vi "YaxisSetup.vi"(8 "Mapping":enum8{"Lin", "Log"}(ring), 9 "HeightAxisBounds":T4, 10 "gnuplotIn":string) -> (2 "gnuplotOut":string)   [LabVIEW 2013]
uses:
  minAndMax.ctl
  AutoManualNumber.ctl
  ticsAndGrids.ctl
  tics.ctl
  grids.ctl
  axisName.ctl
panel:
  in  "Post-setup overrides":string="set ytics format '\\color{g}$%g$' offset 0.8,0\nset ylabel '\\color{g}{$h$ (mm)}' offset 12.8\t# Big offset required as format string makes Ytics look longer than they are"
  in  "HeightTicsAndGrids":T1={"tics"={"ticMin"=10.0, "ticStep"=0.0, "ticMax"=1000.0, "minorDivsPerMajor"=10, "ticSpacing"=enum."Auto Tics", "ticPosition"=enum."Outside, no mirror"}, "Grids"={"Gridlines"=enum."Major and Minor", "Zeroaxis"=enum."No zero axis"}, "Mapping"=enum."Lin"}
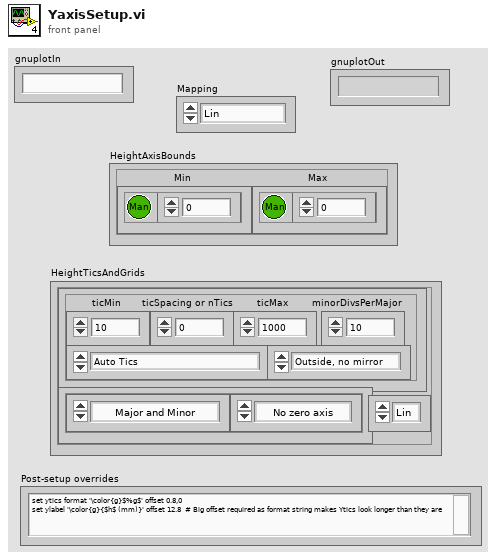
[diagram p1: front panel]
types:
  T1 = typedef "ticsAndGrids.ctl" = cluster{"tics":T2, "Grids":T3, "Mapping":enum8{"Lin", "Log"}}
  T2 = typedef "tics.ctl" = cluster{"ticMin":dbl, "ticStep":dbl, "ticMax":dbl, "minorDivsPerMajor":i32, "ticSpacing":enum16{"Auto Tics", "Fixed spacing", "Fixed Minimum and Spacing", "Start, Spacing and Maximum", "Approx n Tics (rounded)"}, "ticPosition":enum16{"Inside, no mirror", "Inside, mirrored", "Outside, no mirror", "Outside, mirrored", "Invisible"}}
  T3 = typedef "grids.ctl" = cluster{"Gridlines":enum16{"No grids", "Major grid", "Minor grid", "Major and Minor"}, "Zeroaxis":enum16{"No zero axis", "Show zero axis"}}
  T4 = typedef "minAndMax.ctl" = cluster{"Min":T5, "Max":T5}
  T5 = typedef "AutoManualNumber.ctl" = cluster{"Auto":bool, "Value":dbl}
  T6 = typedef "axisName.ctl" = string
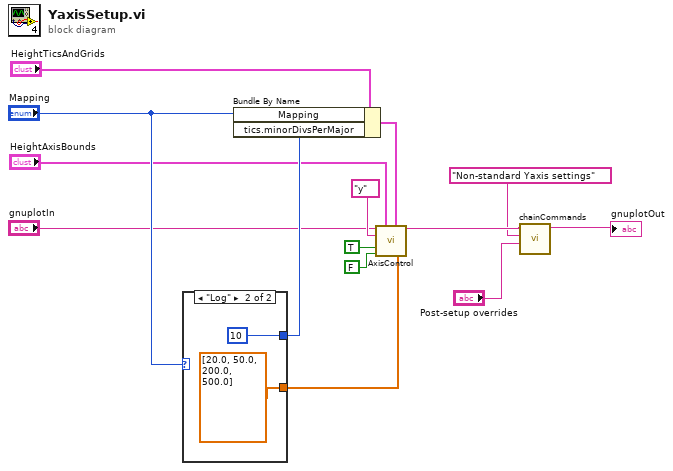
[diagram p0: block diagram]
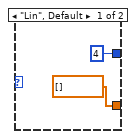
[diagram p2: hidden frame]
diagram:
  n1 = case shown="\"Log\"" "Mapping" {
    tunnel: [dbl[] [] ("AdditionalTics") dbl[] [20.0, 50.0, 200.0, 500.0] ("AdditionalTics")] -> w11
    tunnel: [4 ("minorDivsPerMajor") 10 ("minorDivsPerMajor")] -> w13
    frame "Lin", Default {
    }
    frame "Log" {
    }
  }
  n2 = Bundle By Name(cluster="HeightTicsAndGrids", "Mapping"="Mapping", "tics.minorDivsPerMajor"=w13) -> (w9:T1)
  n3 = call "AxisControl.vi"("String in"="gnuplotIn", "AxisBounds"="HeightAxisBounds", "ticsAndGrids"=w9, "Axis"=T6 "y", "ShowNumbers?"=TRUE, "ShowLabel?"=FALSE ("Set?"), "AdditionalTics"=w11) -> ("String out"=w4:string)  [unwired: 7 in, 1 out]
  n4 = call "chainCommands.vi"("Command"="Post-setup overrides", "Comments"="Non-standard Yaxis settings", "StringIn"=w4) -> ("StringOut"=→"gnuplotOut":string)  [unwired: 8 in]
